vi "opencv.vi"() -> ()   [LabVIEW 2020]
uses:
  <vilib>/vision/Image Controls.llb/IMAQ Image.ctl
panel:
  in  "erosion":u8
  in  "threshold":u8
  out "Processed Image":T1
  in  "stop":bool
  in  "Process Button":bool
  in  "Path":path=path "C:/Users/maxmi/OneDrive/文件/images/original/0.bmp"
  out "Image Processed":T1(plugin-control) caption="Image_merged"
  out "Image":T1(plugin-control)
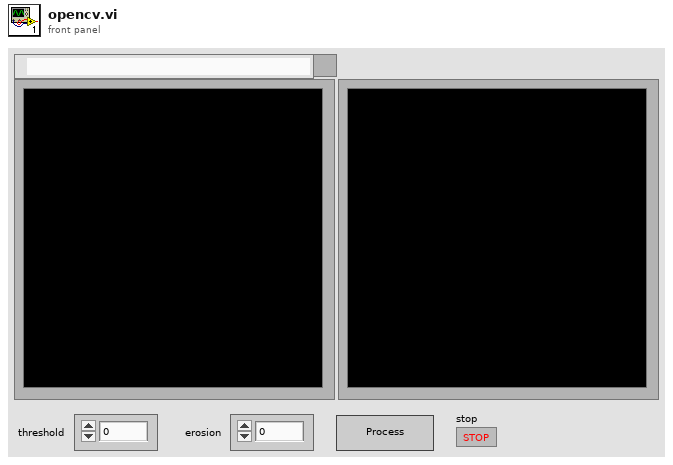
[diagram p1: front panel]
types:
  T1 = typedef "IMAQ Image.ctl" = refnum<image>
  T2 = typedef "Image Type" = u32
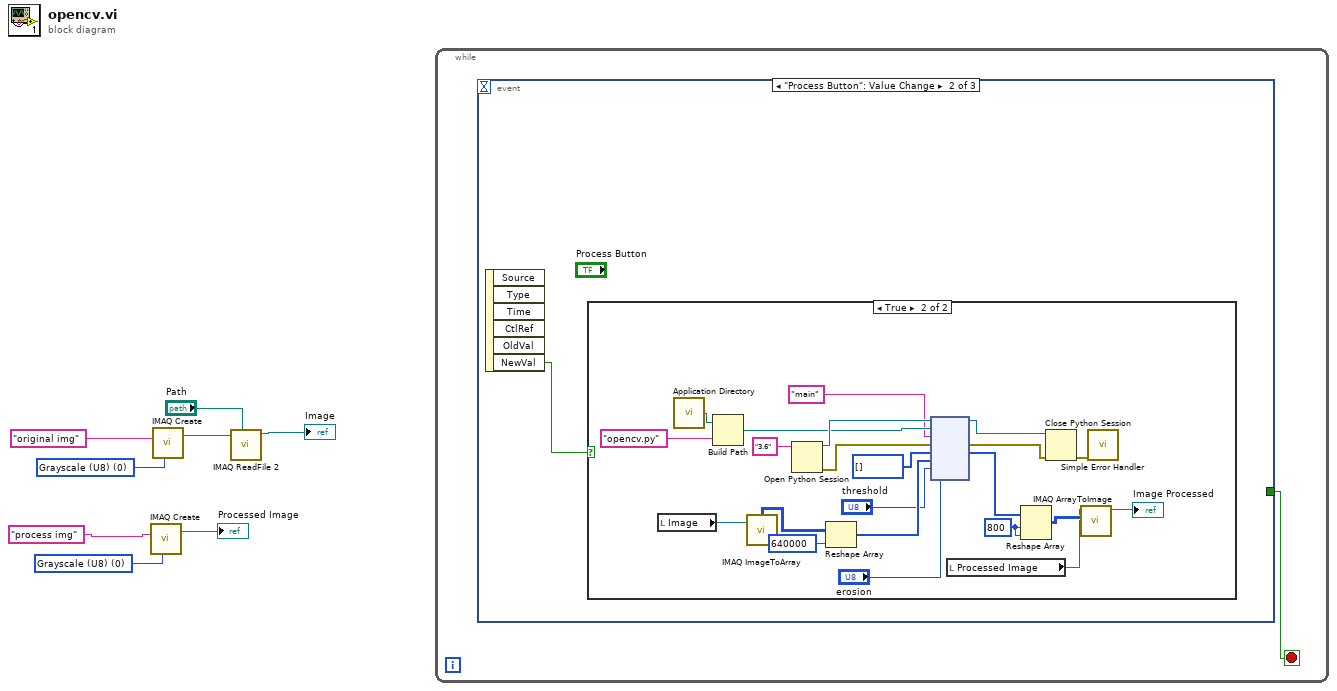
[diagram p0: block diagram]
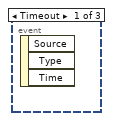
[diagram p2: hidden frame]
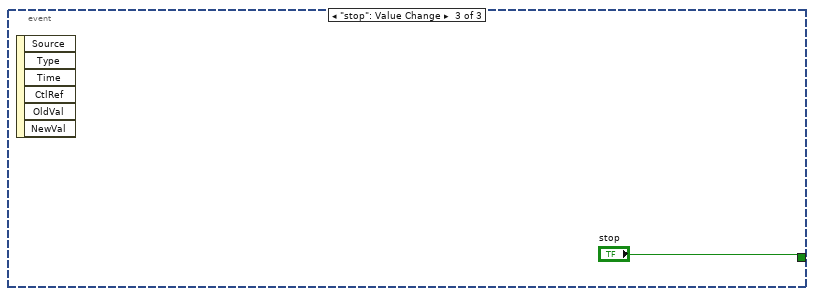
[diagram p4: hidden frame]
diagram:
  w2 = T2 0 items=["Grayscale (U8)", "Grayscale (I16)", "Grayscale (SGL)", "Complex (CSG)", "RGB (U32)", "HSL (U32)", "RGB (U64)", "Grayscale (U16)"] ("Image Type")
  w7 = T2 0 items=["Grayscale (U8)", "Grayscale (I16)", "Grayscale (SGL)", "Complex (CSG)", "RGB (U32)", "HSL (U32)", "RGB (U64)", "Grayscale (U16)"] ("Image Type")
  n1 = call "IMAQ Create"("Image Name"="process img", "Image Type"=w2) -> ("New Image"=→"Processed Image":T1)  [unwired: 2 in, 2 out]
  n2 = call "IMAQ Create"("Image Name"="original img", "Image Type"=w7) -> ("New Image"=w6:T1)  [unwired: 2 in, 2 out]
  n3 = call "IMAQ ReadFile 2"("File Path"="Path", "Image"=w6) -> ("Image Out"=→"Image":T1)  [unwired: 5 in, 4 out]
  n4 = while {
    stop <- w9 stop-if-true
    n5 = event shown="[1] \"Process Button\": Value Change" {
      selector: _ -> [_ _ _]
      dyn-events: _ -> [_ _ _]
      timeout: _ -> [_ _ _]
      tunnel: [_ _ "stop"] -> w9
      event Timeout {
        n6 = event-data() -> ()  [unwired: 1 in, 3 out]
      }
      event "Process Button": Value Change {
        n7 = event-data() -> ("NewVal"=w10:bool)  [unwired: 1 in, 5 out]
        n8 = case shown="True" w10 {
          frame False {
          }
          frame True {
            w16 = 800 ("dimension size")
            n9 = local read "Image"() -> (w21:T1)
            n10 = call <vilib>:"Application Directory.vi"() -> ("Application Directory"=w29:path)
            n11 = Build Path(base path=w29, name or relative path="opencv.py") -> (appended path=w26:path)
            n12 = call "IMAQ ImageToArray"("Image"=w21) -> ("Image Pixels (U8)"=w20:u8[][])  [unwired: 3 in, 4 out]
            n13 = Open Python Session(python version="3.6") -> (session out=w27:refnum<k35>, error out=w28:errorcluster)  [unwired: 2 in]
            n14 = Reshape Array(w20, 640000 ("dimension size")) -> (w18:u8[])
            n15 = node(w27, w26, "main" ("함수 이름"), w28, u8[] [], w18, "threshold", "erosion") -> (w32:refnum<k35>, w31:errorcluster, w17:u8[])  [unwired: 3 in, 2 out]
            n16 = local read "Processed Image"() -> (w13:T1)
            n17 = Reshape Array(w17, w16, w16) -> (w15:u8[][])
            n18 = Close Python Session(session in=w32, error in=w31) -> (11:w30:errorcluster)
            n19 = call "IMAQ ArrayToImage"("Image Pixels (U8)"=w15, "Image"=w13) -> ("Image Out"=→"Image Processed":T1)  [unwired: 8 in, 1 out]
            n20 = call <vilib>:"Simple Error Handler.vi"("error in (no error)"=w30) -> ()  [unwired: 4 in, 5 out]
          }
        }
      }
      event "stop": Value Change {
        n21 = event-data() -> ()  [unwired: 1 in, 6 out]
      }
    }
  }
